vi "CodigoLabView 3.3.vi"() -> (11 "Releb 2":bool)   [LabVIEW 2025]
uses:
  <vilib>/Utility/NIReport.llb/Report Type.ctl
  <vilib>/Instr/_visa.llb/VISA Configure Serial Port (Instr).vi
  <vilib>/addons/_office/excel.llb/Excel Easy Table (str).vi
  <vilib>/Utility/NIReport.llb/NI_report.lvclass
  <vilib>/addons/_office/NI_ReportGenerationToolkit.lvlib
  <vilib>/Utility/NIReport.llb/NI_ReportGenerationCore.lvlib
  <vilib>/Utility/NIReport.llb/Excel/NI_Excel.lvclass
panel:
  out "Histograma V":dbl[](graph)
  out "Histograma 4":dbl[](graph)
  out "Histograma 3":dbl[](graph)
  out "Histograma 2":dbl[](graph)
  out "Histograma 1":dbl[](graph)
  in  "file (use dialog)":path
  out "decimal integer string":string
  in  "?":bool
  in  "file (use dialog) 2":path
  out "Presionado":bool
  in  "RUTA DE REGISTRO":path
  out "Reloj Pot 4":dbl(knob) scale=0.0..100.0
  out "Reloj Pot 3":dbl(knob) scale=0.0..100.0
  out "Reloj Pot 2":dbl(knob) scale=0.0..100.0
  out "R ON 4":bool
  out "R ON 3":bool
  out "R ON 2":bool
  out "?":string
  out "R ON 1":bool
  out "TENSIÓN DE LÍNEA":dbl(knob) scale=100.0..300.0
  out "Reloj Pot 1":dbl(knob) scale=0.0..100.0
  out "Releb 4":bool
  out "Relea 4":bool
  out "Rele 4":bool
  out "TOMACORRIENTE 4":bool
  out "Estado 4":string
  in  "Relé N°4":bool
  out "Potencia 4":string
  out "Releb 3":bool
  out "Relea 3":bool
  out "Rele 3":bool
  out "TOMACORRIENTE 3":bool
  out "Estado 3":string
  out "Potencia 3":string
  in  "Relé N°3":bool
  out "Relea 2":bool
  out "Rele 2":bool
  out "TOMACORRIENTE 2":bool
  out "Estado 2":string
  out "Potencia 2":string
  in  "Relé N°2":bool
  out "Releb 1":bool
  out "Relea 1":bool
  out "Rele 1":bool
  out "TOMACORRIENTE 1":bool
  out "Estado 1":string
  out "Potencia 1":string
  in  "Relé N°1":bool
  in  "PUERTO DE COMUNICACIÓN":refnum<visa-resource-name>
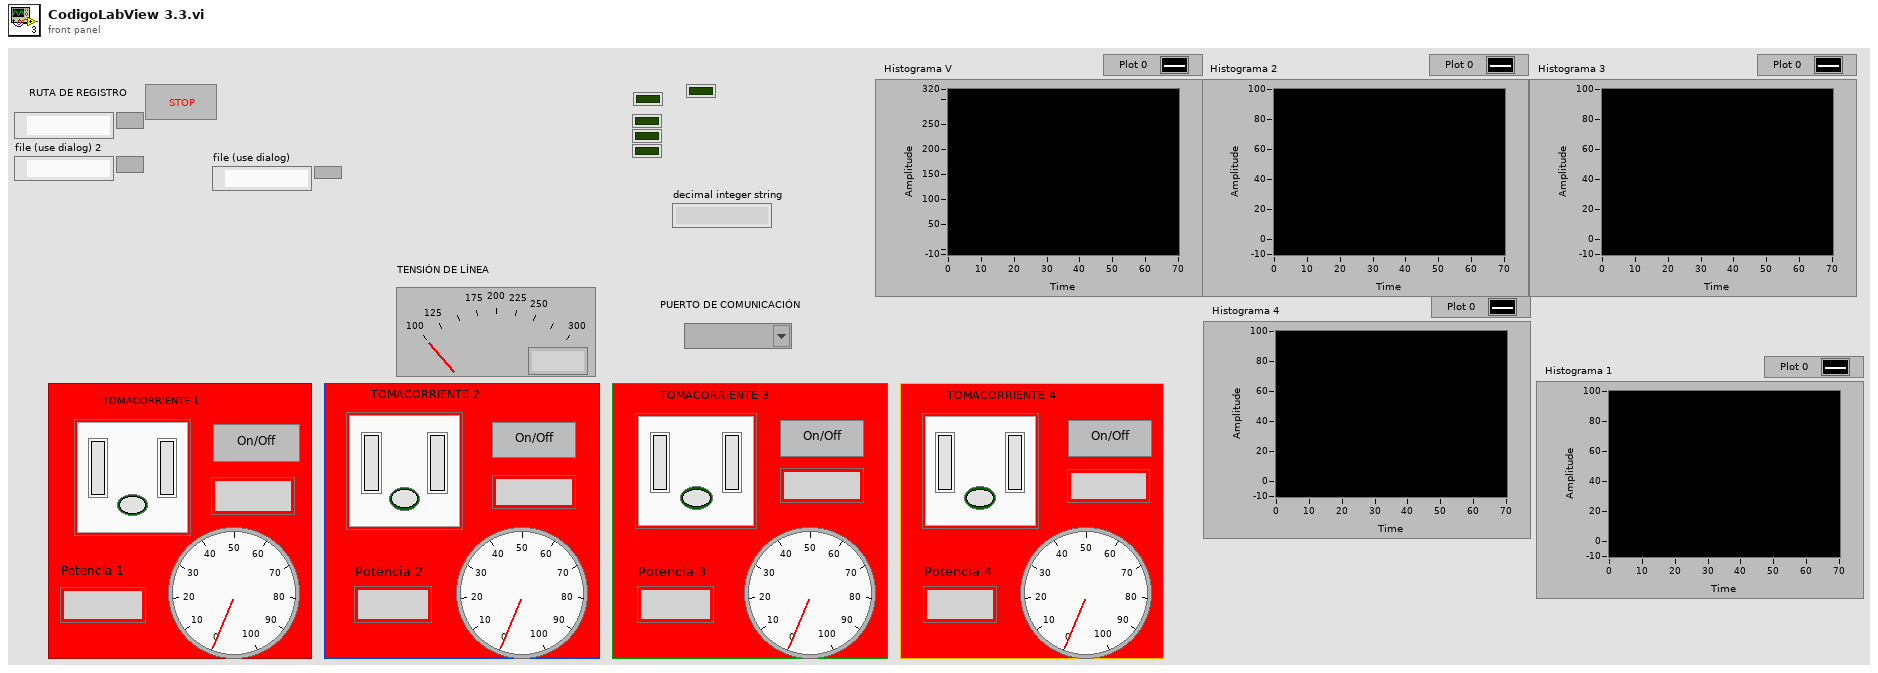
[diagram p1: front panel]
types:
  T1 = typedef "NI_ReportGenerationCore.lvlib/Report Type.ctl" = enum16{"HTML", "Word", "Excel"}
  T2 = cluster{"W1":string, "W2":string, "W3":string, "W4":string, "V":string}
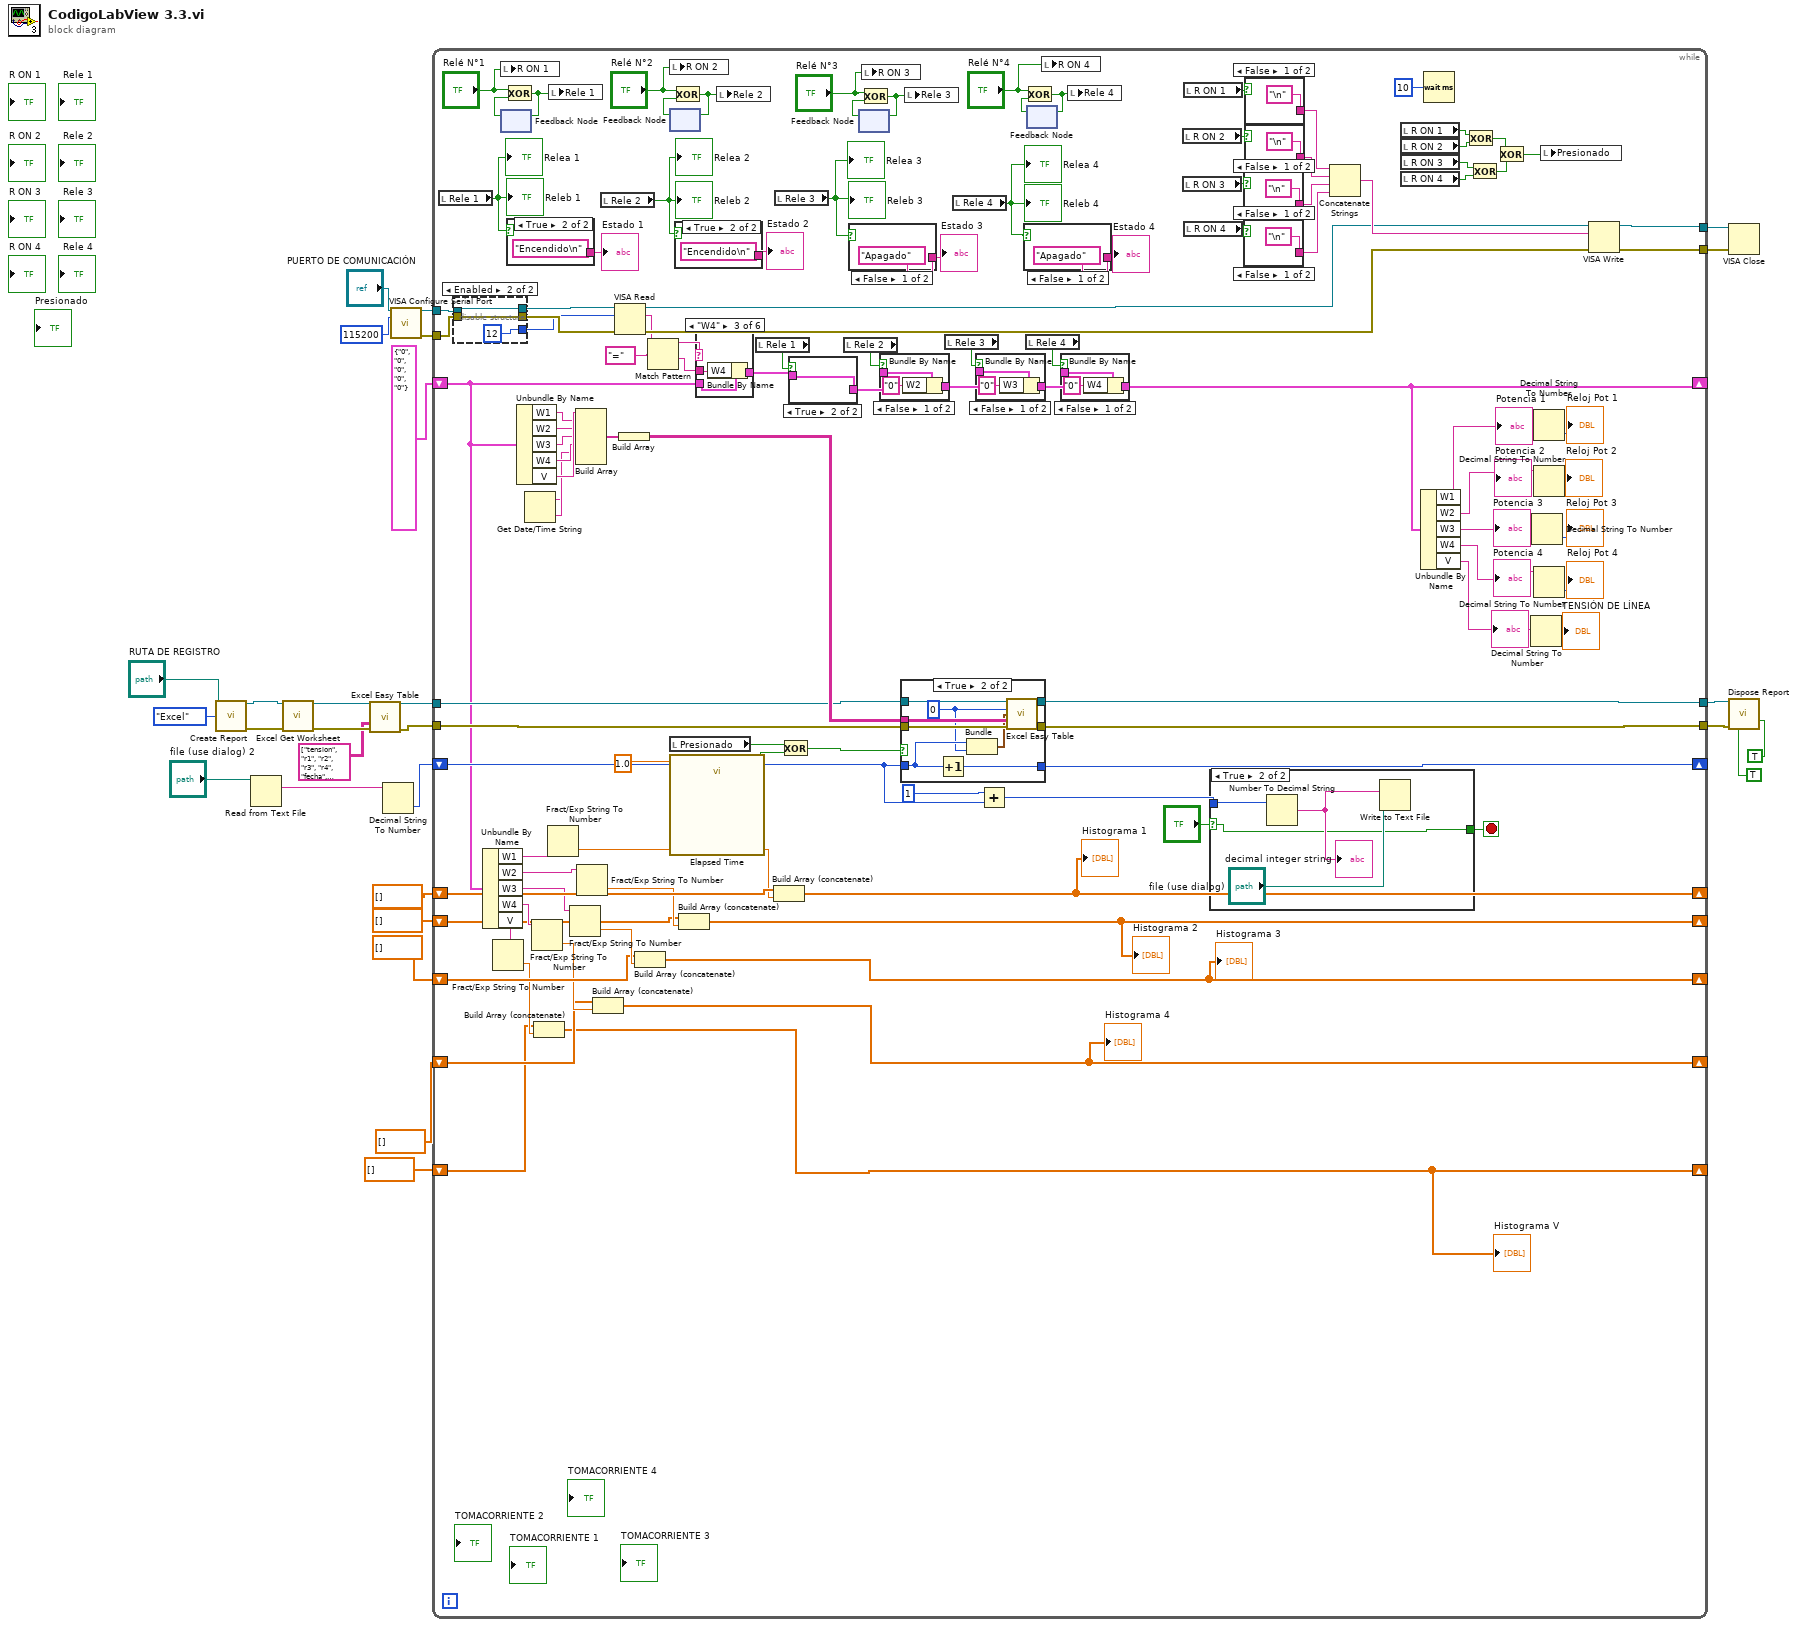
[diagram p0: block diagram]
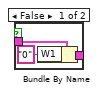
[diagram p5: hidden frame]
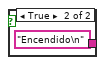
[diagram p8: hidden frame]
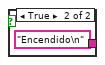
[diagram p9: hidden frame]
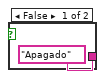
[diagram p10: hidden frame]
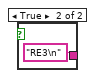
[diagram p11: hidden frame]
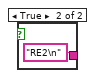
[diagram p12: hidden frame]
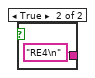
[diagram p13: hidden frame]
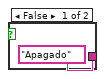
[diagram p14: hidden frame]
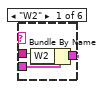
[diagram p15: hidden frame]
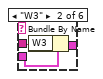
[diagram p16: hidden frame]
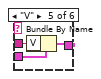
[diagram p18: hidden frame]
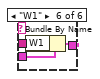
[diagram p19: hidden frame]
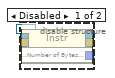
[diagram p20: hidden frame]
diagram:
  n1 = call <vilib>:"Create Report.vi"("report type"=Report_Type."Excel", "template (empty)"="RUTA DE REGISTRO") -> ("report out"=w17:refnum<class "NI_report.lvclass">, "error out"=w16:errorcluster)  [unwired: 12 in]
  n2 = Read from Text File(file (use dialog)="file (use dialog) 2") -> (text=w8:string)  [unwired: 3 in, 3 out]
  n3 = call <vilib>:"Excel Get Worksheet.vi"("report in"=w17, "error in (no error)"=w16) -> ("report out"=w15:refnum<class "NI_report.lvclass">, "error out"=w14:errorcluster)  [unwired: 12 in]
  n4 = call-poly <vilib>:"Excel Easy Table.vi"("report in"=w15, "text data"=string[][] [["tension", "r1", "r2", "r3", "r4", "fecha", "hora"]], "error in (no error)"=w14) -> ("report out"=w12:refnum<class "NI_report.lvclass">, "error out"=w11:errorcluster)  [unwired: 8 in, 3 out]
  n5 = Decimal String To Number(string=w8) -> (number=w6:i32)  [unwired: 2 in, 1 out]
  n6 = call-poly "VISA Configure Serial Port"("VISA resource name"="PUERTO DE COMUNICACIÓN", "baud rate (9600)"=u32 115200) -> ("VISA resource name out"=w28:refnum<visa-resource-name>, "error out"=w25:errorcluster)  [unwired: 12 in]
  n7 = while {
    tunnel: w28 -> [w141]
    tunnel: w25 -> [w140]
    shift-right: [w50] -> _
    shift-left: T2 {"W1"="0", "W2"="0", "W3"="0", "W4"="0", "V"="0"} -> [w45]
    tunnel: [w105] -> w23
    tunnel: [w104] -> w22
    shift-right: [w60] -> _
    shift-left: w6 -> [w51]
    tunnel: w12 -> [w70]
    tunnel: w11 -> [w69]
    tunnel: [w62] -> w10
    tunnel: [w61] -> w9
    shift-right: [w48] -> _
    shift-left: dbl[] [] ("array") -> [w49]
    shift-right: [w38] -> _
    shift-left: dbl[] [] ("array") -> [w39]
    shift-right: [w31] -> _
    shift-left: dbl[] [] ("array") -> [w36]
    shift-right: [w30] -> _
    shift-left: dbl[] [] ("array") -> [w34]
    shift-right: [w29] -> _
    shift-left: dbl[] [] ("array") -> [w32]
    stop <- w52 stop-if-true
    n8 = local read "Rele 1"() -> (w131:bool)
    "Releb 1" <- w131
    "Relea 1" <- w131
    n9 = disable-structure shown="Enabled" {
      disable-tunnel: w141 -> [w208 w211]
      disable-tunnel: w140 -> [w207 w210]
      disable-tunnel: [w206 w211] -> w103
      disable-tunnel: [w205 u32 12 ("Bytes at Port")] -> w101
      disable-tunnel: [w204 w210] -> w102
      frame Disabled {
        n10 = property class="Instr"(reference=w208, error in=w207) -> (reference out=w206:refnum<visa-resource-name>, error out=w204:errorcluster, "Serial Settings:Number of Bytes at Serial Port"=w205:u32)
      }
      frame Enabled {
      }
    }
    n11 = Unbundle By Name(w45) -> ("W1"=w46:string, "W2"=w44:string, "W3"=w43:string, "W4"=w42:string, "V"=w41:string)
    n12 = Fract/Exp String To Number(string=w41) -> (number=w33:dbl)  [unwired: 3 in, 1 out]
    n13 = local write "R ON 1"("Relé N°1") -> ()
    n14 = feedback #1() -> (w135:bool)  [unwired: 1 in]
    n15 = Exclusive Or(1:w135, 2:"Relé N°1") -> (0:w132:bool)
    n16 = feedback-in #1(w132) -> ()
    n17 = case shown="True" w131 {
      tunnel: ["Apagado" "Encendido\n"] -> w134
      frame False {
      }
      frame True {
      }
    }
    "Estado 1" <- w134
    n18 = Unbundle By Name(w45) -> ("W1"=w79:string, "W2"=w78:string, "W3"=w77:string, "W4"=w76:string, "V"=w80:string)
    n19 = Get Date/Time String() -> (date string=w74:string, time string=w75:string)  [unwired: 3 in]
    n20 = Fract/Exp String To Number(string=w42) -> (number=w35:dbl)  [unwired: 3 in, 1 out]
    n21 = Build Array (concatenate)(w32, w33) -> (w29:dbl[])
    "Histograma V" <- w29
    n22 = Fract/Exp String To Number(string=w46) -> (number=w47:dbl)  [unwired: 3 in, 1 out]
    n23 = local write "Rele 1"(w132) -> ()
    n24 = Fract/Exp String To Number(string=w43) -> (number=w37:dbl)  [unwired: 3 in, 1 out]
    n25 = Build Array(w80, w79, w78, w77, w76, w74, w75) -> (w72:string[])
    n26 = Fract/Exp String To Number(string=w44) -> (number=w40:dbl)  [unwired: 3 in, 1 out]
    n27 = Build Array (concatenate)(w34, w35) -> (w30:dbl[])
    "Histograma 4" <- w30
    n28 = local read "Rele 2"() -> (w123:bool)
    "Releb 2" <- w123
    "Relea 2" <- w123
    n29 = VISA Read(VISA resource name=w103, byte count=w101, error in (no error)=w102) -> (VISA resource name out=w100:refnum<visa-resource-name>, read buffer=w98:string, error out=w99:errorcluster)  [unwired: 1 out]
    n30 = Build Array(w72) -> (w73:string[][])
    n31 = Build Array (concatenate)(w36, w37) -> (w31:dbl[])
    "Histograma 3" <- w31
    n32 = Match Pattern(string=w98, regular expression="=") -> (before substring=w137:string, after substring=w107:string)  [unwired: 1 in, 2 out]
    n33 = local write "R ON 2"("Relé N°2") -> ()
    n34 = feedback #2() -> (w125:bool)  [unwired: 1 in]
    n35 = local read "Presionado"() -> (w56:bool)
    n36 = call "Elapsed Time"("Time Target (s)"=1.0) -> ("Time has Elapsed"=w58:bool)  [unwired: 11 in, 7 out]
    n37 = Exclusive Or(1:w125, 2:"Relé N°2") -> (0:w124:bool)
    n38 = feedback-in #2(w124) -> ()
    n39 = case shown="True" w123 {
      tunnel: ["Apagado" "Encendido\n"] -> w122
      frame False {
      }
      frame True {
      }
    }
    "Estado 2" <- w122
    n40 = Build Array (concatenate)(w39, w40) -> (w38:dbl[])
    "Histograma 2" <- w38
    n41 = case shown="\"W4\"" w137 {
      tunnel: w107 -> [w188 w191 w194 _ w198 w201]
      tunnel: w45 -> [w190 w193 w196 w197 w200 w203]
      tunnel: [w189 w192 w195 w197 w199 w202] -> w88
      frame "W2" {
        n42 = Bundle By Name(cluster=w190, "W2"=w188) -> (w189:T2)
      }
      frame "W3" {
        n43 = Bundle By Name(cluster=w193, "W3"=w191) -> (w192:T2)
      }
      frame "W4" {
        n44 = Bundle By Name(cluster=w196, "W4"=w194) -> (w195:T2)
      }
      frame "False", Default {
      }
      frame "V" {
        n45 = Bundle By Name(cluster=w200, "V"=w198) -> (w199:T2)
      }
      frame "W1" {
        n46 = Bundle By Name(cluster=w203, "W1"=w201) -> (w202:T2)
      }
    }
    n47 = local write "Rele 2"(w124) -> ()
    n48 = local read "Rele 1"() -> (w81:bool)
    n49 = Build Array (concatenate)(w49, w47) -> (w48:dbl[])
    "Histograma 1" <- w48
    n50 = local read "Rele 3"() -> (w118:bool)
    "Relea 3" <- w118
    "Releb 3" <- w118
    n51 = Exclusive Or(1:w58, 2:w56) -> (0:w57:bool)
    n52 = case shown="True" w81 {
      tunnel: w88 -> [w163 w165]
      tunnel: [w162 w165] -> w87
      frame False {
        n53 = Bundle By Name(cluster=w163, "W1"="0") -> (w162:T2)
      }
      frame True {
      }
    }
    n54 = local read "Rele 2"() -> (w82:bool)
    n55 = case shown="False" w118 {
      tunnel: ["Apagado" "Encendido\n"] -> w114
      frame False {
      }
      frame True {
      }
    }
    "Estado 3" <- w114
    n56 = feedback #3() -> (w120:bool)  [unwired: 1 in]
    n57 = Exclusive Or(1:w120, 2:"Relé N°3") -> (0:w119:bool)
    n58 = feedback-in #3(w119) -> ()
    n59 = local write "R ON 3"("Relé N°3") -> ()
    n60 = case shown="False" w82 {
      tunnel: w87 -> [w167 w169]
      tunnel: [w166 w169] -> w86
      frame False {
        n61 = Bundle By Name(cluster=w167, "W2"="0") -> (w166:T2)
      }
      frame True {
      }
    }
    n62 = case shown="True" w57 {
      tunnel: w73 -> [_ w157]
      tunnel: w69 -> [w148 w156]
      tunnel: [w147 w155] -> w62
      tunnel: [w148 w154] -> w61
      tunnel: w70 -> [w147 w153]
      tunnel: w51 -> [w146 w152]
      tunnel: [w146 w151] -> w60
      frame False {
      }
      frame True {
        w149 = 0 ("iteration")
        n63 = Increment(x=w152) -> (x+1=w151:i32)
        n64 = Bundle(w152, "iteration"=w149) -> (w150:cluster{i32, "iteration":i32})  [unwired: 1 in]
        n65 = call-poly <vilib>:"Excel Easy Table.vi"("report in"=w153, "iteration"=w149, "start (0, 0)"=w150, "text data"=w157, "error in (no error)"=w156) -> ("report out"=w155:refnum<class "NI_report.lvclass">, "error out"=w154:errorcluster)  [unwired: 6 in, 3 out]
      }
    }
    n66 = local write "Rele 3"(w119) -> ()
    n67 = local read "Rele 3"() -> (w83:bool)
    n68 = local read "Rele 4"() -> (w113:bool)
    "Relea 4" <- w113
    "Releb 4" <- w113
    n69 = case shown="False" w83 {
      tunnel: w86 -> [w159 w161]
      tunnel: [w158 w161] -> w85
      frame False {
        n70 = Bundle By Name(cluster=w159, "W3"="0") -> (w158:T2)
      }
      frame True {
      }
    }
    n71 = Add(x=1, y=w51) -> (x+y=w54:i32)
    n72 = case shown="False" w113 {
      tunnel: ["Apagado" "Encendido\n"] -> w112
      frame False {
      }
      frame True {
      }
    }
    "Estado 4" <- w112
    n73 = local read "Rele 4"() -> (w84:bool)
    n74 = feedback #4() -> (w116:bool)  [unwired: 1 in]
    n75 = Exclusive Or(1:w116, 2:"Relé N°4") -> (0:w115:bool)
    n76 = feedback-in #4(w115) -> ()
    n77 = local write "R ON 4"("Relé N°4") -> ()
    n78 = case shown="False" w84 {
      tunnel: w85 -> [w171 w173]
      tunnel: [w170 w173] -> w50
      frame False {
        n79 = Bundle By Name(cluster=w171, "W4"="0") -> (w170:T2)
      }
      frame True {
      }
    }
    n80 = local write "Rele 4"(w115) -> ()
    n81 = local read "R ON 2"() -> (w128:bool)
    n82 = local read "R ON 3"() -> (w127:bool)
    n83 = local read "R ON 1"() -> (w130:bool)
    n84 = local read "R ON 4"() -> (w129:bool)
    n85 = case shown="True" "?" {
      selector: "?" -> [_ w142]
      tunnel: w54 -> [_ w143]
      tunnel: [_ w142] -> w52
      frame False {
      }
      frame True {
        n86 = Number To Decimal String(number=w143) -> (decimal integer string=w144:string)  [unwired: 1 in]
        "decimal integer string" <- w144
        n87 = Write to Text File(file (use dialog)="file (use dialog)", text=w144) -> ()  [unwired: 2 in, 3 out]
      }
    }
    n88 = case shown="False" w127 {
      tunnel: ["\n" "RE3\n"] -> w109
      frame False {
      }
      frame True {
      }
    }
    n89 = case shown="False" w129 {
      tunnel: ["\n" "RE4\n"] -> w110
      frame False {
      }
      frame True {
      }
    }
    n90 = case shown="False" w130 {
      tunnel: ["\n" "RE1\n"] -> w136
      frame False {
      }
      frame True {
      }
    }
    n91 = case shown="False" w128 {
      tunnel: ["\n" "RE2\n"] -> w111
      frame False {
      }
      frame True {
      }
    }
    n92 = Concatenate Strings(w136, w111, w109, w110) -> (w106:string)
    n93 = local read "R ON 1"() -> (w68:bool)
    n94 = local read "R ON 2"() -> (w67:bool)
    n95 = local read "R ON 3"() -> (w65:bool)
    n96 = local read "R ON 4"() -> (w66:bool)
    n97 = Unbundle By Name(w50) -> ("W1"=w97:string, "W2"=w92:string, "W3"=w91:string, "W4"=w90:string, "V"=w89:string)
    "Potencia 1" <- w97
    "?" <- w89
    "Potencia 2" <- w92
    "Potencia 3" <- w91
    "Potencia 4" <- w90
    n98 = Wait (ms)(milliseconds to wait=u32 10) -> ()  [unwired: 1 out]
    n99 = Exclusive Or(1:w67, 2:w68) -> (0:w63:bool)
    n100 = Exclusive Or(1:w66, 2:w65) -> (0:w64:bool)
    n101 = Exclusive Or(1:w64, 2:w63) -> (0:w59:bool)
    n102 = Decimal String To Number(string=w89) -> (number=→"TENSIÓN DE LÍNEA":i32)  [unwired: 2 in, 1 out]
    n103 = Decimal String To Number(string=w91) -> (number=→"Reloj Pot 3":i32)  [unwired: 2 in, 1 out]
    n104 = Decimal String To Number(string=w97) -> (number=→"Reloj Pot 1":i32)  [unwired: 2 in, 1 out]
    n105 = Decimal String To Number(string=w92) -> (number=→"Reloj Pot 2":i32)  [unwired: 2 in, 1 out]
    n106 = Decimal String To Number(string=w90) -> (number=→"Reloj Pot 4":i32)  [unwired: 2 in, 1 out]
    n107 = local write "Presionado"(w59) -> ()
    n108 = VISA Write(VISA resource name=w100, write buffer=w106, error in (no error)=w99) -> (VISA resource name out=w105:refnum<visa-resource-name>, error out=w104:errorcluster)  [unwired: 1 out]
  }
  n109 = VISA Close(VISA resource name=w23, error in (no error)=w22) -> ()  [unwired: 1 out]
  n110 = call-dynamic "Dispose Report.vi"("report in"=w10, "save changes? (F)"=TRUE, "error in (no error)"=w9, "close report? (T)"=TRUE) -> ()  [unwired: 11 in, 1 out]
